vi "Read Write Edge Image (SubVI).vi"   [LabVIEW 2015]
uses:
  <vilib>/rvi/Emulation/niFpgaEmulationIsFPGAContextNoSignature.vi
  <vilib>/rvi/Emulation/niFpgaSctlEmulationGetInTimedLoop.vi
  <vilib>/rvi/errors/niFpgaSetErrorForExecOnDevCompSimple.vi
  <vilib>/rvi/eio/common/nirviEmuReportErrorAndStop.vi
  <vilib>/rvi/DataTransferAndStorage/Container/Common/niFpgaContainerGetUniqueNameForEmu.vi
  <vilib>/rvi/FIFO/Fifo_Resource/nirvififoEmulationSetSize.vi
  <vilib>/rvi/FIFO/Fifo_Resource/nirviFifoEmulationQueueMgr.vi
  <instcachedir>/0/nirviFifoEmulationQueueMgr_E5CAEC123FF24DC58D834DCA3CDAA9B5.lvgen/nirviFifoEmulationQueueMgr_E5CAEC123FF24DC58D834DCA3CDAA9B5_004.vi
  <vilib>/Utility/error.llb/Clear Errors.vi
  <vilib>/rvi/FIFO/Fifo_Resource/nirvififoEmulationCreateLock.vi
  <vilib>/rvi/Emulation/niFpgaProcessEmulError.vi
  <vilib>/rvi/FIFO/Fifo_Resource/nirvififoEmulationObtainLock.vi
  <vilib>/rvi/FIFO/Fifo_Resource/nirvififoEmulationReleaseLock.vi
  <vilib>/rvi/occurrence/nirviWaitOnOccurrenceBase.vi
  <vilib>/rvi/errors/nirviReportUnexpectedCaseInternalError.vi
  <vilib>/rvi/errors/nirviReportUnexpectedCaseInternalError (U32).vi
  <vilib>/rvi/Memory/Memory_Emulation/nirvimemoryFastEmulation.vi
  <vilib>/rvi/Memory/Memory_Emulation/nirvimemoryEmulation.vi
  <instcachedir>/0/nirviFifoEmulationQueueMgr_E5CAEC123FF24DC58D834DCA3CDAA9B5.lvgen/nirviFifoEmulationQueueMgr_E5CAEC123FF24DC58D834DCA3CDAA9B5_001.vi
  <vilib>/rvi/FIFO/Fifo_Resource/nirvififoEmulationDetermineInputValidOut.vi
  <vilib>/rvi/DataTransferAndStorage/Container/XNode/niFpgaContainer.xnode
  <vilib>/rvi/FIFO/Fifo_Resource/nirvififoEmulationRead.vi
  <vilib>/rvi/FIFO/Fifo_Resource/nirvififoEmulationWrite.vi
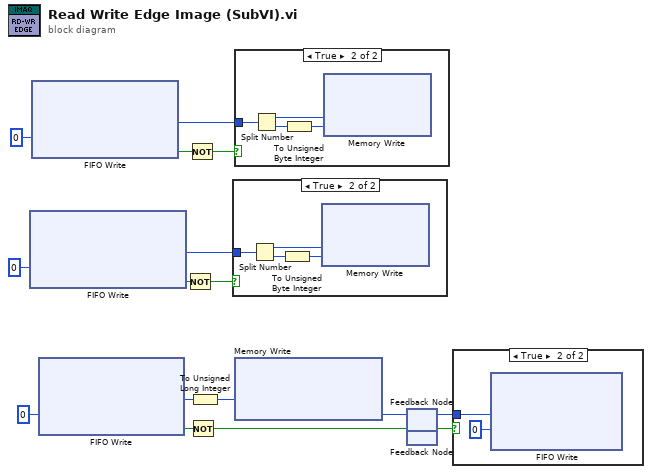
[diagram p0: block diagram]
diagram:
  n1 = xnode ("FIFO Write")("Timeout"=0) -> ("Element"=w10:u64, "Timed Out?"=w12:bool)  [unwired: 1 in, 1 out]
  n2 = xnode ("FIFO Write")("Timeout"=0) -> ("Element"=w7:u64, "Timed Out?"=w1:bool)  [unwired: 1 in, 1 out]
  n3 = xnode ("FIFO Write")("Timeout"=0) -> ("Element"=w5:u64, "Timed Out?"=w4:bool)  [unwired: 1 in, 1 out]
  n4 = Not(x=w12) -> (.not. x?=w9:bool)
  n5 = Not(x=w1) -> (.not. x?=w8:bool)
  n6 = Not(x=w4) -> (.not. x?=w14:bool)
  n7 = To Unsigned Long Integer(number=w5) -> (unsigned 32bit integer=w6:u32)
  n8 = case shown="True" w9 {
    tunnel: w10 -> [_ w20]
    frame False {
    }
    frame True {
      n9 = Split Number(x=w20) -> (hi(x)=w19:u32, lo(x)=w18:u32)
      n10 = To Unsigned Byte Integer(number=w18) -> (unsigned 8bit integer=w17:u8)
      n11 = xnode ("Memory Write")("Address"=w19, "Data"=w17) -> ()  [unwired: 1 in, 1 out]
    }
  }
  n12 = case shown="True" w8 {
    tunnel: w7 -> [_ w24]
    frame False {
    }
    frame True {
      n13 = Split Number(x=w24) -> (hi(x)=w23:u32, lo(x)=w22:u32)
      n14 = To Unsigned Byte Integer(number=w22) -> (unsigned 8bit integer=w21:u8)
      n15 = xnode ("Memory Write")("Address"=w23, "Data"=w21) -> ()  [unwired: 1 in, 1 out]
    }
  }
  n16 = xnode ("Memory Write")("Address"=w6) -> ("Data"=w13:u8)  [unwired: 1 in, 1 out]
  n17 = feedback #1() -> (w15:u8)  [unwired: 1 in]
  n18 = feedback-in #1(w13) -> ()
  n19 = feedback #2() -> (w16:bool)  [unwired: 1 in]
  n20 = feedback-in #2(w14) -> ()
  n21 = case shown="True" w16 {
    tunnel: w15 -> [_ w25]
    frame False {
    }
    frame True {
      n22 = xnode ("FIFO Write")("Element"=w25, "Timeout"=0) -> ()  [unwired: 1 in, 2 out]
    }
  }
